vi "Get File Path for Load and Save.vi"(8 "error in (no error)":errorcluster, 10 "Save/Load":bool, 11 "Scheduler in":refnum<class "Scheduler.lvclass">) -> (0 "error out":errorcluster, 3 "Scheduler out":refnum<class "Scheduler.lvclass">)   [LabVIEW 2020, in "Scheduler.lvlib" / "Scheduler.lvclass"]
uses:
  Scheduler.lvclass
  Scheduler Consumer Case Selector.ctl
  TALOS/TALOS_PPL.lvlibp/Father of all uServices/Father of all uServices/Father of all uServices.lvclass
  TALOS/TALOS_PPL.lvlibp
  C:/Users/aegis/Documents/CIRCUS/TALOS/TALOS_PPL.lvlibp/Father of all uServices/Father of all uServices/Father of all uServices.lvclass
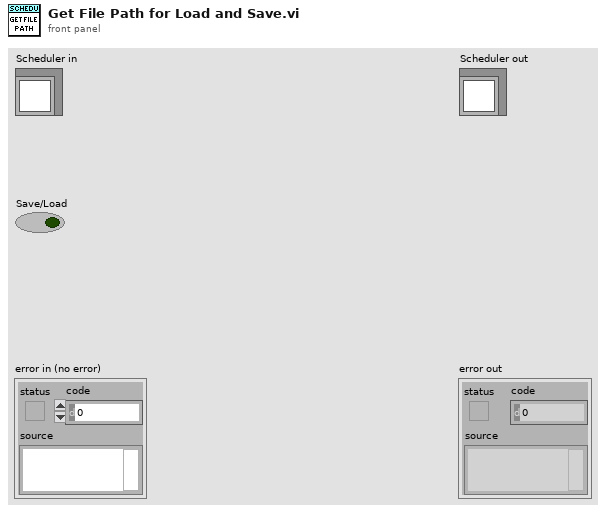
[diagram p1: front panel]
types:
  T1 = typedef "Scheduler.lvlib/Scheduler.lvclass/Scheduler Consumer Case Selector.ctl" = enum16{"Add SBlock", "Update GUI", "Move SBlock", "Select SBlock", "Update Cont.", "Load", "Save", "Reset", "Send to Tamer", "Edit SBlock", "Duplicate SBlock", "Delete SBlock", "Update SBlock", "Init", "Split/Combine Schedules", "Reschedule", "Load Parameters"}
  T2 = enum16{"open", "replace", "create", "open or create", "replace or create", "replace or create with confirmation"}
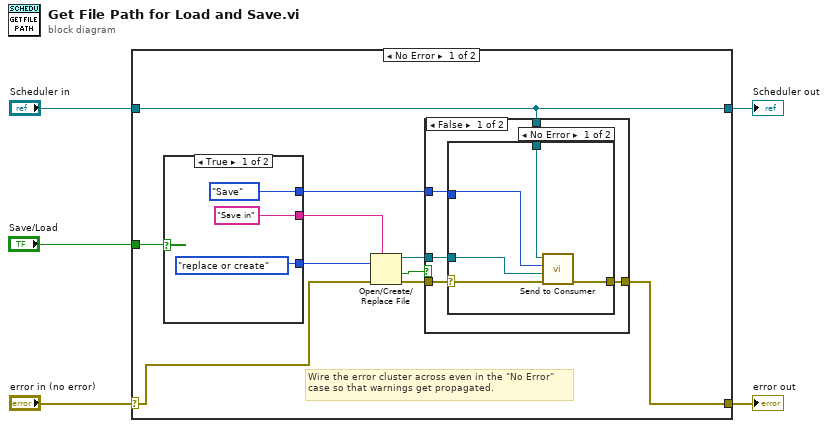
[diagram p0: block diagram]
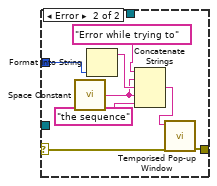
[diagram p2: hidden frame]
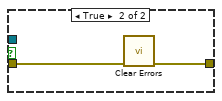
[diagram p3: hidden frame]
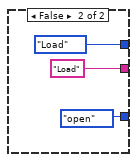
[diagram p4: hidden frame]
diagram:
  n1 = case shown="No Error" "error in (no error)" {
    selector: "error in (no error)" -> [w12 w43]
    tunnel: [w10 w43] -> w4
    tunnel: [w8 w42] -> w2
    tunnel: "Scheduler in" -> [w8 w42]
    tunnel: "Save/Load" -> [w15 _]
    frame No Error {
      # "Wire the error cluster across even in the \"No Error\"\ncase so that warnings get propagated."
      n2 = case shown="True" w15 {
        tunnel: ["Save in" ("prompt") "Load" ("prompt")] -> w14
        tunnel: [T2."replace or create" ("operation (0:open)") T2."open" ("operation (0:open)")] -> w13
        tunnel: [Scheduler_Consumer_Case_Selector."Save" ("Shifter Panel Consumer Case Selector") Scheduler_Consumer_Case_Selector."Load" ("Shifter Panel Consumer Case Selector")] -> w6
        frame True {
        }
        frame False {
        }
      }
      n3 = Open/Create/Replace File(error in=w12, prompt=w14, operation (0:open)=w13) -> (refnum out=w9:refnum<file>, cancelled=w11:bool, error out=w7:errorcluster)  [unwired: 3 in]
      n4 = case shown="False" w11 {
        tunnel: w7 -> [w16 w35]
        tunnel: [w19 w34] -> w10
        tunnel: w9 -> [w17 _]
        tunnel: w8 -> [w20 _]
        tunnel: w6 -> [w18 _]
        frame False {
          n5 = case shown="No Error" w16 {
            selector: w16 -> [w22 w33]
            tunnel: w20 -> [w21 _]
            tunnel: [w25 w32] -> w19
            tunnel: w18 -> [w24 w31]
            tunnel: w17 -> [w23 _]
            frame No Error {
              n6 = call "Send to Consumer.vi"("error in (no error)"=w22, "Data"=w23, "Case ID"=w24, "uService Template in"=w21) -> ("error out"=w25:errorcluster)  [unwired: 6 in, 1 out]
            }
            frame Error {
              n7 = call <vilib>:"Space Constant.vi"() -> ("String"=w28:string)
              n8 = Format Into String(w31) -> (resulting string=w29:string)  [unwired: 3 in, 1 out]
              n9 = Concatenate Strings("Error while trying to" ("Text"), w28, w29, w28, "the sequence" ("string")) -> (w26:string)
              n10 = call "Temporised Pop-up Window.vi"("error in (no error)"=w33, "Text"=w26) -> ("error out"=w32:errorcluster)  [unwired: 9 in]
            }
          }
        }
        frame True {
          n11 = call <vilib>:"Clear Errors.vi"("error in (no error)"=w35) -> ("error out"=w34:errorcluster)  [unwired: 5 in, 1 out]
        }
      }
    }
    frame Error {
    }
  }
  "error out" <- w4
  "Scheduler out" <- w2
